vi "add-exp-eventSD.vi"(0 "Exp name":string, 1 "Update graphs of exp":refnum<user-event>, 2 "add exp":bool, 3 "cluster in":T2={"Experiments groups"=[], "Kinetics"=[], "Spectrum"=[], "GRAPH EXPERIMENTAL DATA"=[], "kinetics plot names"=[], "spectra plot names"=[], "group"=0, "exp selected"=0, "# exp"=0, "error out"={"status"=FALSE, "code"=0, "source"=""}, "FromToWave"={"FromWave"=0.0, "ToWave"=0.0}, "GRAPH EXPERIMENTAL DATA ref"=refnum, "timedelays"=[0.0, 0.0, 0.0, 0.0, 0.0, 0.0, 0.0, 0.06019061100911815, 0.0521779104562645, 0.045231877429679615, 0.03921051490799832, 0.033990728811568754, 0.029465811603150715, 0.025543260876973825, 0.02214288834180205, 0.01919518054014414, 0.016639877791965713, 0.014424742312398925, 0.012504490320209958, 0.010839866306230088, 0.009396840537117498, 0.008145913389103785, 0.00706151229029317, 0.006121468943269439, 0.005306566140927374, 0.004600144911132549, 0.003987763959109073, 0.0034569044455719407, 0.00299671406541447, 0.0025977851951783253, 0.0022519625739982996, 0.00195217658646366, 0.0016922987392150965, 0.0014670163768006634, 0.0012717240756200802, 0.0011024294957352762, 0.0009556717658856477, 0.0008284507332614981, 0.0007181656316962257, 0.0006225619144775864, 0.0005396851648867825, 0.00046784114226338394, 0.0004055611468220084, 0.0003515719951773376, 0.00030476999279031153, 0.00026419837125694315, 0.00022902772919263772, 0.0001985390768670671, 0.0001721091379728629, 0.00014919760805372974, 0.00012933610911736794], "wavelengths"=[0.0, 0.0, 0.0, 0.0, 0.0, 0.0, 0.0, 0.06019061100911815, 0.0521779104562645, 0.045231877429679615, 0.03921051490799832, 0.033990728811568754, 0.029465811603150715, 0.025543260876973825, 0.02214288834180205, 0.01919518054014414, 0.016639877791965713, 0.014424742312398925, 0.012504490320209958, 0.010839866306230088, 0.009396840537117498, 0.008145913389103785, 0.00706151229029317, 0.006121468943269439, 0.005306566140927374, 0.004600144911132549, 0.003987763959109073, 0.0034569044455719407, 0.00299671406541447, 0.0025977851951783253, 0.0022519625739982996, 0.00195217658646366, 0.0016922987392150965, 0.0014670163768006634, 0.0012717240756200802, 0.0011024294957352762, 0.0009556717658856477, 0.0008284507332614981, 0.0007181656316962257, 0.0006225619144775864, 0.0005396851648867825, 0.00046784114226338394, 0.0004055611468220084, 0.0003515719951773376, 0.00030476999279031153, 0.00026419837125694315, 0.00022902772919263772, 0.0001985390768670671, 0.0001721091379728629, 0.00014919760805372974, 0.00012933610911736794], "Experiment"=refnum, "Commentaires exp"=refnum, "FromToDelay"={"FromDelay"=0.0, "ToDelay"=0.0}}, 4 "Commentaires exp":string, 5 "Bounds":T1) -> (7 "cluster out":T2={"Experiments groups"=[], "Kinetics"=[], "Spectrum"=[], "GRAPH EXPERIMENTAL DATA"=[], "kinetics plot names"=[], "spectra plot names"=[], "group"=0, "exp selected"=0, "# exp"=0, "error out"={"status"=FALSE, "code"=0, "source"=""}, "FromToWave"={"FromWave"=0.0, "ToWave"=0.0}, "GRAPH EXPERIMENTAL DATA ref"=refnum, "timedelays"=[0.0, 0.0, 0.0, 0.0, 0.0, 0.0, 0.0, 0.06019061100911815, 0.0521779104562645, 0.045231877429679615, 0.03921051490799832, 0.033990728811568754, 0.029465811603150715, 0.025543260876973825, 0.02214288834180205, 0.01919518054014414, 0.016639877791965713, 0.014424742312398925, 0.012504490320209958, 0.010839866306230088, 0.009396840537117498, 0.008145913389103785, 0.00706151229029317, 0.006121468943269439, 0.005306566140927374, 0.004600144911132549, 0.003987763959109073, 0.0034569044455719407, 0.00299671406541447, 0.0025977851951783253, 0.0022519625739982996, 0.00195217658646366, 0.0016922987392150965, 0.0014670163768006634, 0.0012717240756200802, 0.0011024294957352762, 0.0009556717658856477, 0.0008284507332614981, 0.0007181656316962257, 0.0006225619144775864, 0.0005396851648867825, 0.00046784114226338394, 0.0004055611468220084, 0.0003515719951773376, 0.00030476999279031153, 0.00026419837125694315, 0.00022902772919263772, 0.0001985390768670671, 0.0001721091379728629, 0.00014919760805372974, 0.00012933610911736794], "wavelengths"=[0.0, 0.0, 0.0, 0.0, 0.0, 0.0, 0.0, 0.06019061100911815, 0.0521779104562645, 0.045231877429679615, 0.03921051490799832, 0.033990728811568754, 0.029465811603150715, 0.025543260876973825, 0.02214288834180205, 0.01919518054014414, 0.016639877791965713, 0.014424742312398925, 0.012504490320209958, 0.010839866306230088, 0.009396840537117498, 0.008145913389103785, 0.00706151229029317, 0.006121468943269439, 0.005306566140927374, 0.004600144911132549, 0.003987763959109073, 0.0034569044455719407, 0.00299671406541447, 0.0025977851951783253, 0.0022519625739982996, 0.00195217658646366, 0.0016922987392150965, 0.0014670163768006634, 0.0012717240756200802, 0.0011024294957352762, 0.0009556717658856477, 0.0008284507332614981, 0.0007181656316962257, 0.0006225619144775864, 0.0005396851648867825, 0.00046784114226338394, 0.0004055611468220084, 0.0003515719951773376, 0.00030476999279031153, 0.00026419837125694315, 0.00022902772919263772, 0.0001985390768670671, 0.0001721091379728629, 0.00014919760805372974, 0.00012933610911736794], "Experiment"=refnum, "Commentaires exp"=refnum, "FromToDelay"={"FromDelay"=0.0, "ToDelay"=0.0}})   [LabVIEW 2015]
uses:
  controls/control-cluster.ctl
  Classes/Experiments_group.lvclass
  Classes/Experiment.lvclass
  globalVarSD.vi
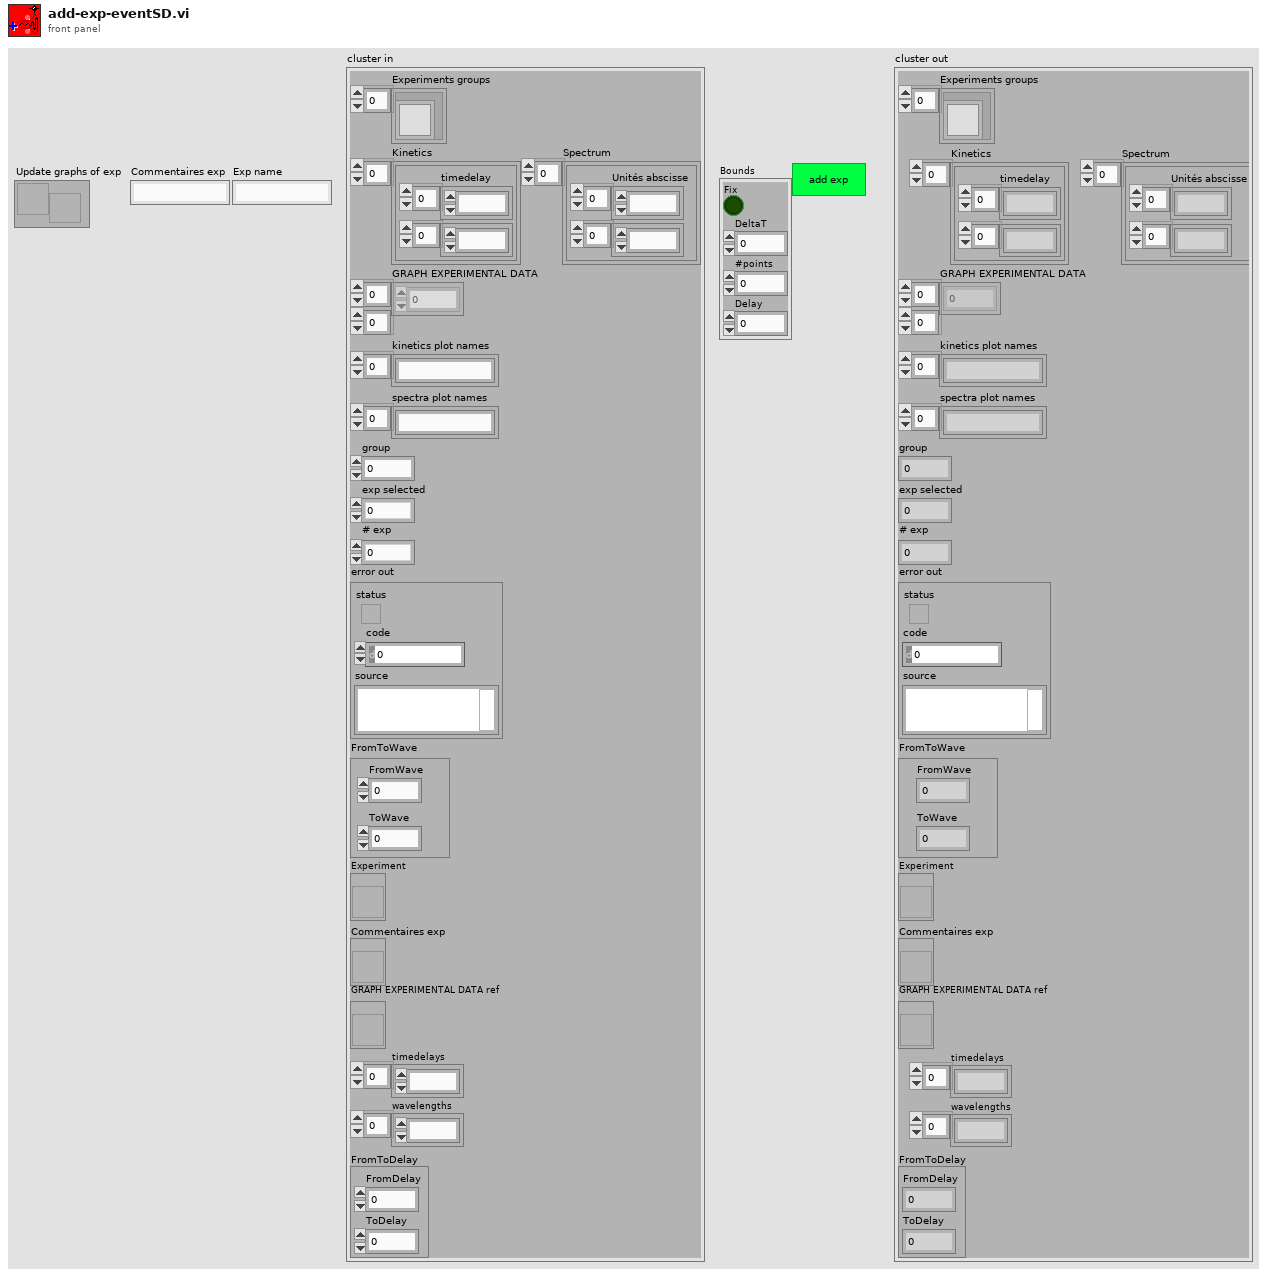
[diagram p1: front panel]
types:
  T1 = cluster{"Fix":bool, "DeltaT":dbl, "#points":i32, "Delay":dbl}
  T2 = typedef "control-cluster.ctl" = cluster{"Experiments groups":refnum<class "Experiments_group.lvclass">[], "Kinetics":cluster{"timedelay":dbl[], dbl[]}[], "Spectrum":cluster{"Unités abscisse":dbl[], dbl[]}[], "GRAPH EXPERIMENTAL DATA":dbl[][], "kinetics plot names":string[], "spectra plot names":string[], "group":i32, "exp selected":i32, "# exp":i32, "error out":errorcluster, "FromToWave":cluster{"FromWave":dbl, "ToWave":dbl}, "GRAPH EXPERIMENTAL DATA ref":refnum<vi>, "timedelays":dbl[], "wavelengths":dbl[], "Experiment":refnum<vi>, "Commentaires exp":refnum<vi>, "FromToDelay":cluster{"FromDelay":dbl, "ToDelay":dbl}}
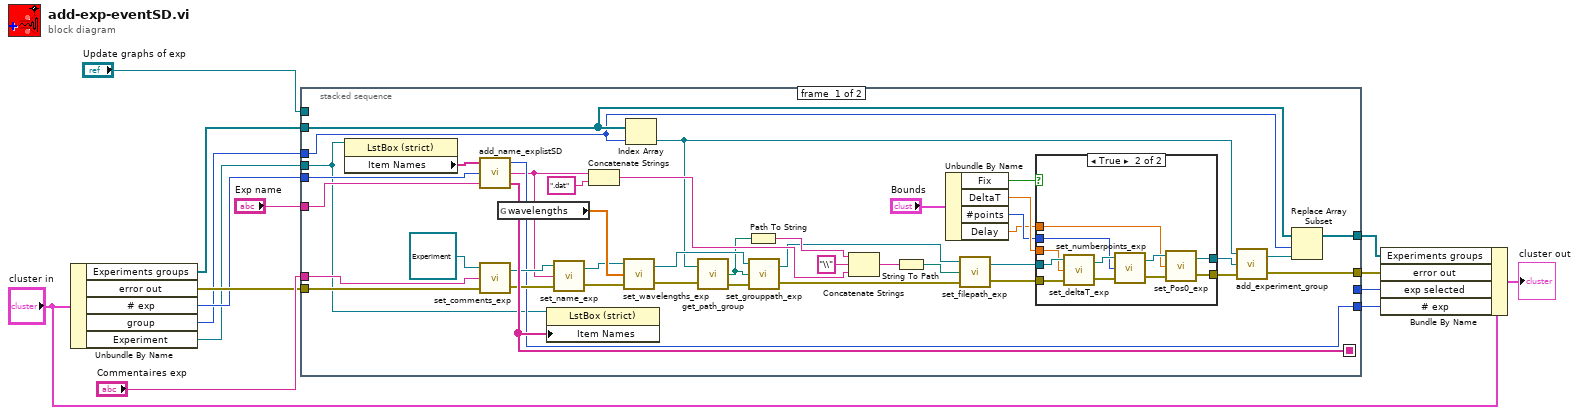
[diagram p0: block diagram]
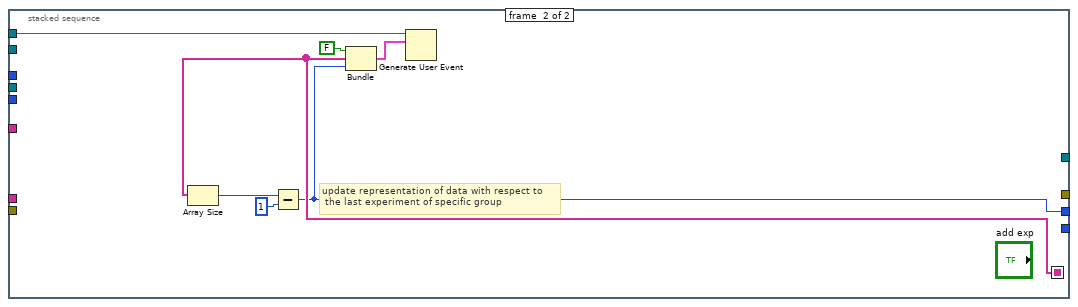
[diagram p3: hidden frame]
diagram:
  n1 = Unbundle By Name("cluster in") -> ("Experiments groups"=w8:refnum<class "Experiments_group.lvclass">[], "error out"=w7:errorcluster, "# exp"=w4:i32, "group"=w2:i32, "Experiment"=w1:refnum<vi>)
  n2 = stacked-sequence {
    seq-local: [w53 _] -> [_ w72]
    tunnel: [w54 _] -> w9
    tunnel: [w34 _] -> w6
    tunnel: "Update graphs of exp" -> [_ w74]
    tunnel: w8 -> [w51 _]
    tunnel: w7 -> [w46 _]
    tunnel: [_ w71] -> w5
    tunnel: w4 -> [w45 _]
    tunnel: [w44 _] -> w3
    tunnel: "Exp name" -> [w43 _]
    tunnel: "Commentaires exp" -> [w42 _]
    tunnel: w2 -> [w41 _]
    tunnel: w1 -> [w40 _]
    frame #0 {
      n3 = property on="Property Node" class="LstBox (strict)"(reference=w40) -> ("Item Names"=w55:string[])  [unwired: 1 in, 2 out]
      n4 = call "add_name_explistSD.vi"("Exp name"=w43, "exp #"=w45, "Item Names in"=w55) -> ("Item Names out"=w53:string[], "name out"=w22:string, "Numeric"=w44:i32)
      n5 = call-dynamic "set_comments_exp.vi"("error in (no error)"=w46, "Comments"=w42, "Experiment.lvclass in"=refnum<class "Experiment.lvclass"> refnum ("Experiment.lvclass")) -> ("error out"=w48:errorcluster, "Experiment.lvclass out"=w50:refnum<class "Experiment.lvclass">)
      n6 = global read "globalVarSD.vi" "wavelengths"() -> (w52:dbl[])
      n7 = property on="Property Node" class="LstBox (strict)"(reference=w40, "Item Names"=w53) -> ()  [unwired: 1 in, 2 out]
      n8 = call-dynamic "set_name_exp.vi"("error in (no error)"=w48, "Exp name"=w22, "Experiment.lvclass in"=w50) -> ("error out"=w47:errorcluster, "Experiment.lvclass out"=w49:refnum<class "Experiment.lvclass">)
      n9 = Concatenate Strings(w22, ".dat" ("string")) -> (w24:string)
      n10 = call-dynamic "set_wavelengths_exp.vi"("error in (no error)"=w47, "wavelengths"=w52, "Experiment.lvclass in"=w49) -> ("error out"=w37:errorcluster, "Experiment.lvclass out"=w39:refnum<class "Experiment.lvclass">)
      n11 = Index Array(array=w51, index=w41) -> (element=w21:refnum<class "Experiments_group.lvclass">)
      n12 = call-dynamic "get_path_group.vi"("Experiments_group.lvclass in"=w21, "error in (no error)"=w37) -> ("Path"=w15:path, "error out"=w38:errorcluster)  [unwired: 1 out]
      n13 = Path To String(path=w15) -> (string=w26:string)
      n14 = call-dynamic "set_grouppath_exp.vi"("error in (no error)"=w38, "GroupPath"=w15, "Experiment.lvclass in"=w39) -> ("error out"=w17:errorcluster, "Experiment.lvclass out"=w19:refnum<class "Experiment.lvclass">)
      n15 = Concatenate Strings(w26, "\\" ("string"), w24) -> (w25:string)
      n16 = String To Path(string=w25) -> (path=w20:path)
      n17 = Unbundle By Name("Bounds") -> ("Fix"=w35:bool, "DeltaT"=w30:dbl, "#points"=w29:i32, "Delay"=w28:dbl)
      n18 = call-dynamic "set_filepath_exp.vi"("error in (no error)"=w17, "FilePath"=w20, "Experiment.lvclass in"=w19) -> ("error out"=w16:errorcluster, "Experiment.lvclass out"=w18:refnum<class "Experiment.lvclass">)
      n19 = case shown="True" w35 {
        tunnel: w18 -> [w58 w69]
        tunnel: [w58 w66] -> w32
        tunnel: [w57 w65] -> w31
        tunnel: w16 -> [w57 w62]
        tunnel: w30 -> [_ w61]
        tunnel: w29 -> [_ w60]
        tunnel: w28 -> [_ w59]
        frame False {
        }
        frame True {
          n20 = call-dynamic "set_deltaT_exp.vi"("error in (no error)"=w62, "deltaTlast"=w61, "Experiment.lvclass in"=w69) -> ("error out"=w63:errorcluster, "Experiment.lvclass out"=w68:refnum<class "Experiment.lvclass">)
          n21 = call-dynamic "set_numberpoints_exp.vi"("error in (no error)"=w63, "numberpoints"=w60, "Experiment.lvclass in"=w68) -> ("error out"=w64:errorcluster, "Experiment.lvclass out"=w67:refnum<class "Experiment.lvclass">)
          n22 = call-dynamic "set_Pos0_exp.vi"("error in (no error)"=w64, "Pos0,ps"=w59, "Experiment.lvclass in"=w67) -> ("error out"=w65:errorcluster, "Experiment.lvclass out"=w66:refnum<class "Experiment.lvclass">)
        }
      }
      n23 = call-dynamic "add_experiment_group.vi"("error in (no error)"=w31, "Experiment.lvclass"=w32, "Experiments_group.lvclass in"=w21) -> ("error out"=w34:errorcluster, "Experiments_group.lvclass out"=w33:refnum<class "Experiments_group.lvclass">)
      n24 = Replace Array Subset(array=w51, new element=w33, index=w41) -> (w54:refnum<class "Experiments_group.lvclass">[])
    }
    frame #1 {
      # "update representation of data with respect to\n the last experiment of specific group"
      n25 = Array Size(array=w72) -> (size(s)=w75:i32)
      n26 = Subtract(x=w75, y=1) -> (x-y=w71:i32)
      n27 = Bundle(FALSE, "Item Names out"=w72, w71) -> (w70:cluster{bool, "Item Names out":string[], i32})  [unwired: 1 in]
      n28 = Generate User Event(user event=w74, event data cluster=w70) -> ()  [unwired: 2 in, 2 out]
    }
  }
  n29 = Bundle By Name(cluster="cluster in", "Experiments groups"=w9, "error out"=w6, "exp selected"=w5, "# exp"=w3) -> (→"cluster out":T2)
